vi "Test 1.vi"() -> ()   [LabVIEW 2014]
panel:
  out "concatenated string":string
  out "Error Out":errorcluster
  in  "Error In":errorcluster
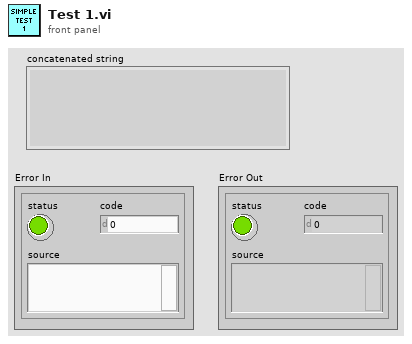
[diagram p1: front panel]
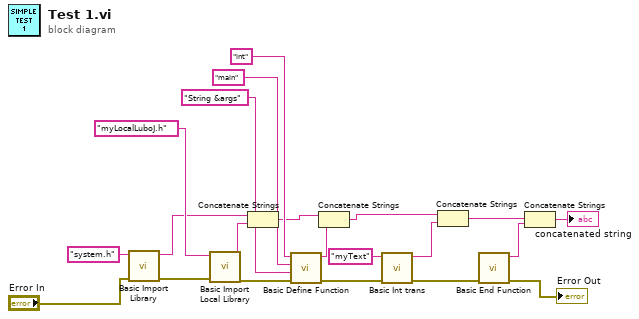
[diagram p0: block diagram]
diagram:
  n1 = call "Basic Import Library.vi"("Error In"="Error In", "system library name"="system.h") -> ("Error Out"=w19:errorcluster, "resulting string"=w12:string)  [unwired: 8 in]
  n2 = call "Basic Import Local Library.vi"("Error In"=w19, "local library name"="myLocalLuboJ.h" ("system library name")) -> ("Error Out"=w17:errorcluster, "resulting string"=w13:string)  [unwired: 8 in]
  n3 = Concatenate Strings(w12, w13) -> (w11:string)
  n4 = call "Basic Define Function.vi"("Error In"=w17, "args"="String &args", "name"="main", "return type"="int") -> ("Error Out"=w6:errorcluster, "resulting string"=w10:string)  [unwired: 6 in]
  n5 = Concatenate Strings(w11, w10) -> (w3:string)
  n6 = call "Basic Int trans.vi"("Error In"=w6, "int variable name"="myText") -> ("Error Out"=w5:errorcluster, "resulting string"=w2:string)  [unwired: 8 in]
  n7 = Concatenate Strings(w3, w2) -> (w1:string)
  n8 = call "Basic End Function.vi"("Error In"=w5) -> ("Error Out"=→"Error Out":errorcluster, "resulting string"=w9:string)  [unwired: 9 in]
  n9 = Concatenate Strings(w1, w9) -> (→"concatenated string":string)
